vi "GetParam.vi"(8 "error in (no error)":errorcluster caption="entrée d'erreur (pas d'erreur)", 11 "Pairwise_distances.lvclass":refnum<class "Pairwise_distances.lvclass">) -> (0 "error out":errorcluster caption="sortie d'erreur", 2 "pairwise_distances":T1={"metric "="euclidean", "n_jobs"="None", "force_all_finite "="True"}, 3 "Pairwise_distances.lvclass":refnum<class "Pairwise_distances.lvclass">)   [LabVIEW 2020, in "Pairwise_distances.lvclass"]
doc: "Get Parameters"
uses:
  Pairwise_distances.lvclass
  Pairwise_distances.lvclass/Pairwise_distances.ctl
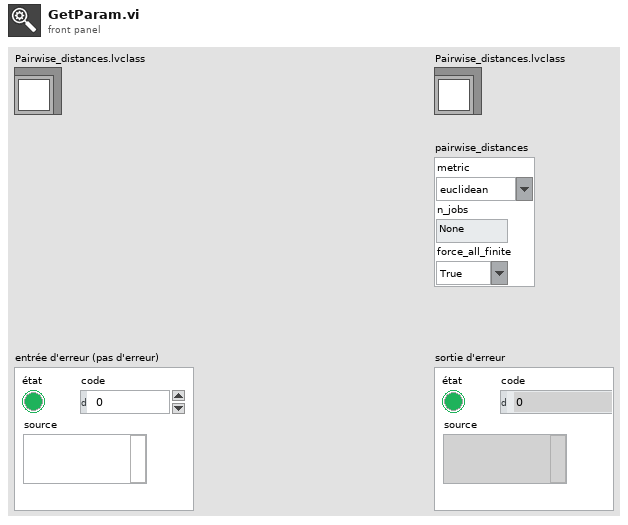
[diagram p1: front panel]
types:
  T1 = cluster{"metric ":string, "n_jobs":string, "force_all_finite ":string}
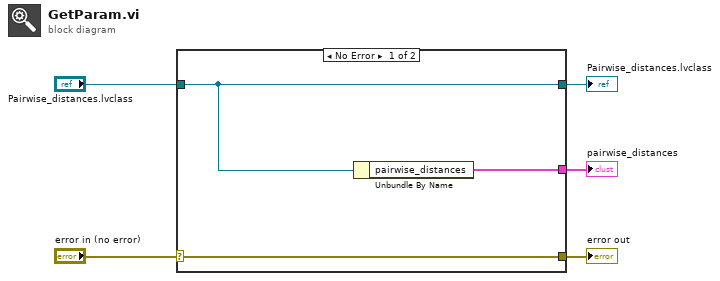
[diagram p0: block diagram]
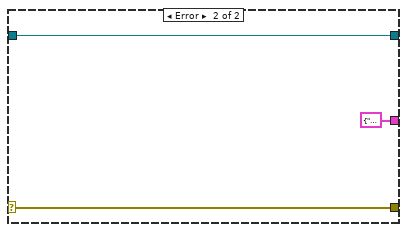
[diagram p2: hidden frame]
diagram:
  n1 = case shown="No Error" "error in (no error)" {
    selector: "error in (no error)" -> [w8 w10]
    tunnel: [w8 w10] -> w4
    tunnel: [w7 w11] -> w2
    tunnel: "Pairwise_distances.lvclass" -> [w7 w11]
    tunnel: [w6 T1 {"metric "="", "n_jobs"="", "force_all_finite "=""} ("pairwise_distances")] -> w1
    frame No Error {
      n2 = Unbundle By Name(w7) -> ("pairwise_distances"=w6:T1)
    }
    frame Error {
    }
  }
  "error out" <- w4
  "Pairwise_distances.lvclass" <- w2
  "pairwise_distances" <- w1
